vi "Save2010.vi"   [LabVIEW 2013]
uses:
  ErrorCodes.ctl
  <vilib>/Heliosphere Research LLC/Advanced Plotting Toolkit/Advanced Plotting Toolkit.lvlib
types:
  T1 = typedef "ErrorCodes.ctl" = u32
  T2 = typedef "Advanced Plotting Toolkit.lvlib/PlotID.ctl" = i32
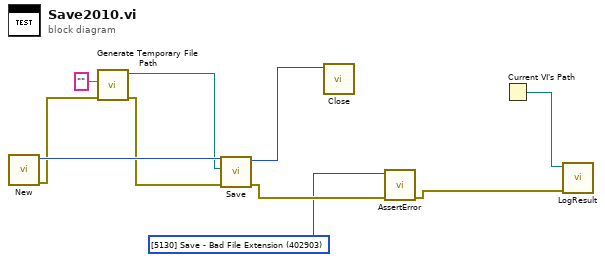
[diagram p0: block diagram]
diagram:
  w1 = T1 402903 items=["[5120] Invalid ID"=402902, "[5110] Failed to Init"=402900, "[5111] Unknown Error"=402901, "[5130] Save - Bad File Extension"=402903, "[5131] Save - General Error"=402904, "[5140] Unsupported (Polar)"=402905, "[5141] Unsupported (Logscale)"=402906, "[5142] Coordinates Not Regular"=402907] ("Expected Error")
  n1 = call <vilib>:"New.vi"() -> ("error out"=w7:errorcluster, "Plot ID"=w8:T2)  [unwired: 10 in]
  n2 = call <vilib>:"Generate Temporary File Path.vi"("error in (no error)"=w7, "Temporary File Extension (tmp)"="") -> ("error out"=w6:errorcluster, "Unique Temporary File Path"=w5:path)  [unwired: 8 in]
  n3 = call <vilib>:"Save.vi"("error in (no error)"=w6, "Path"=w5, "Plot ID In"=w8) -> ("error out"=w3:errorcluster, "Plot ID Out"=w4:T2)  [unwired: 7 in]
  n4 = call <vilib>:"Close.vi"("Plot ID"=w4) -> ()  [unwired: 10 in, 1 out]
  n5 = call "AssertError.vi"("error in (no error)"=w3, "Expected Error"=w1) -> ("error out"=w2:errorcluster)  [unwired: 9 in]
  n6 = Current VI's Path() -> (path=w10:path)
  n7 = call "LogResult.vi"("Test Result"=w2, "VI Path"=w10) -> ()  [unwired: 10 in]
